vi "XIPIN_Concat_2_1.vi"   [LabVIEW 2017]
doc: "Concatenates up to 32 ports into a single port\n------------------------------------\n<b>Need License</b> : No"
uses:
  <vilib>/rvi/XilinxIP/XIPIN_XNode/niFpgaXIPIN.xnode
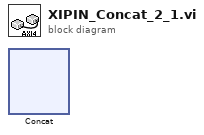
[diagram p0: block diagram]
diagram:
  n1 = xnode ("Concat")() -> ()
